vi "Get Primary Key.vi"(8 "error in (no error)":errorcluster, 10 "Table Name Array":string[](array[string]), 11 "ADODB in":refnum<class "ADODB.lvclass">) -> (0 "error out":errorcluster, 1 "PK Found?":bool[](array[boolean]), 2 "Primary Key Array":T1[](array[typedef]), 3 "ADODB out":refnum<class "ADODB.lvclass">)   [LabVIEW 2020, in "ADODB.lvlib" / "ADODB.lvclass"]
uses:
  ADODB.lvclass
  Database Interfaces/Primary Key Info.ctl
  ADODB.lvclass/ADODB.ctl
  ADODB.lvlib
  <vilib>/addons/database/NI_Database_API.lvlib
  Database Interfaces.lvlib
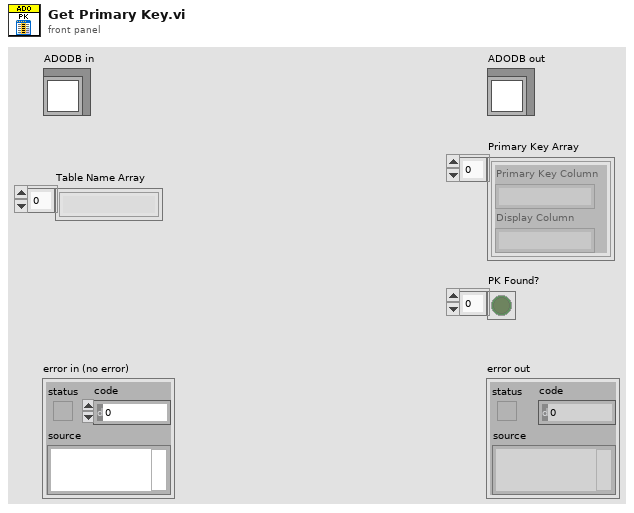
[diagram p1: front panel]
types:
  T1 = typedef "Database Interfaces.lvlib/Primary Key Info.ctl" = cluster{"Primary Key Column":string, "Display Column":string}
  T2 = typedef "NI_Database_API.lvlib/Conn ObjectReference.ctl" = refnum<k1>
  T3 = typedef "NI_Database_API.lvlib/Conn DataMembers.ctl" = cluster{"ADODB._Connection":refnum<k7>, "recordset objects":i32, "command objects":i32}
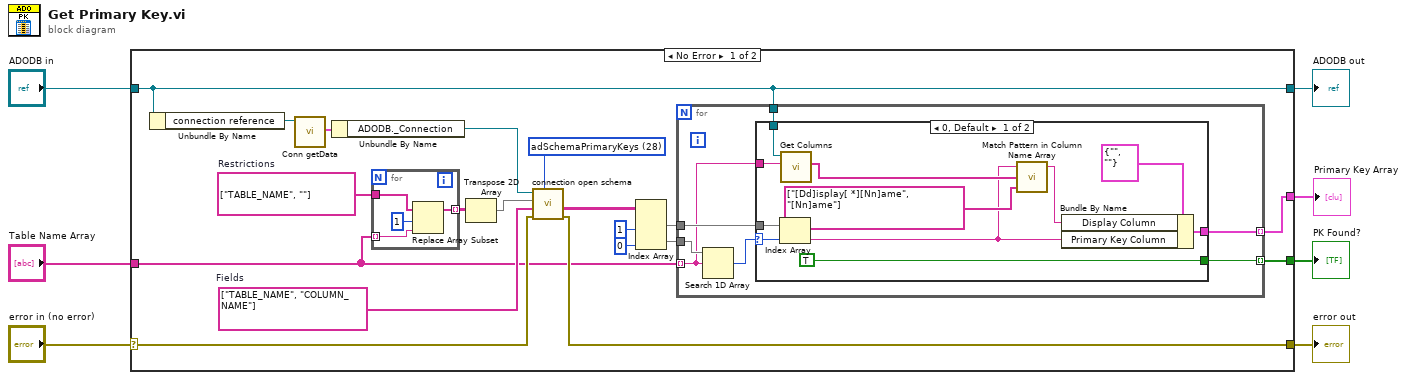
[diagram p0: block diagram]
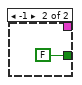
[diagram p2: hidden frame]
diagram:
  n1 = case shown="No Error" "error in (no error)" {
    selector: "error in (no error)" -> [w22 w51]
    tunnel: [w21 w51] -> w6
    tunnel: "ADODB in" -> [w8 w50]
    tunnel: [w8 w50] -> w4
    tunnel: "Table Name Array" -> [w18 _]
    tunnel: [w12 _] -> w1
    tunnel: [w11 _] -> w2
    frame No Error {
      w19 = string[] ["TABLE_NAME", ""]  # Restrictions
      w20 = string[] ["TABLE_NAME", "COLUMN_NAME"]  # Fields
      w23 = 28 items=["adSchemaProviderSpecific"=-1, "adSchemaAsserts"=0, "adSchemaCatalogs"=1, "adSchemaCharacterSets"=2, "adSchemaCollations"=3, "adSchemaColumns"=4, "adSchemaCheckConstraints"=5, "adSchemaConstraintColumnUsage"=6, "adSchemaConstraintTableUsage"=7, "adSchemaKeyColumnUsage"=8, "adSchemaReferentialContraints, adSchemaReferentialConstraints"=9, "adSchemaTableConstraints"=10, "adSchemaColumnsDomainUsage"=11, "adSchemaIndexes"=12, "adSchemaColumnPrivileges"=13, "adSchemaTablePrivileges"=14, "adSchemaUsagePrivileges"=15, "adSchemaProcedures"=16, "adSchemaSchemata"=17, "adSchemaSQLLanguages"=18, "adSchemaStatistics"=19, "adSchemaTables"=20, "adSchemaTranslations"=21, "adSchemaProviderTypes"=22, "adSchemaViews"=23, "adSchemaViewColumnUsage"=24, "adSchemaViewTableUsage"=25, "adSchemaProcedureParameters"=26, "adSchemaForeignKeys"=27, "adSchemaPrimaryKeys"=28, "adSchemaProcedureColumns"=29, "adSchemaDBInfoKeywords"=30, "adSchemaDBInfoLiterals"=31, "adSchemaCubes"=32, "adSchemaDimensions"=33, "adSchemaHierarchies"=34, "adSchemaLevels"=35, "adSchemaMeasures"=36, "adSchemaProperties"=37, "adSchemaMembers"=38, "adSchemaTrustees"=39] ("Schema")
      n2 = Unbundle By Name(w8) -> ("connection reference"=w26:T2)
      n3 = call <vilib>:"Conn getData.vi"("connection reference"=w26) -> ("data"=w25:T3)  [unwired: 3 in, 3 out]
      n4 = Unbundle By Name(w25) -> ("ADODB._Connection"=w24:refnum<k7>)
      n5 = for {
        tunnel: w18 -> [w48] mode=indexing
        tunnel: [w47] -> w10 mode=indexing
        tunnel: w19 -> [w46]
        n6 = Replace Array Subset(array=w46, new element=w48, index=1 ("index (row)")) -> (w47:string[])
      }
      n7 = Transpose 2D Array(2D array=w10) -> (transposed array=w9:string[][])
      n8 = call "connection open schema.vi"("Schema"=w23, "error in (no error)"=w22, "Fields"=w20, "Restrictions"=w9, "ADODB._Connection"=w24) -> ("error out"=w21:errorcluster, "Schema Out"=w17:string[][])  [unwired: 3 in, 2 out]
      n9 = Index Array(array=w17, index (col) #1=1 ("disabled index (col)"), index (col) #2=0 ("index (col)")) -> (element #1=w13:string[], element #2=w14:string[])  [unwired: 2 in]
      n10 = for {
        tunnel: w18 -> [w28] mode=indexing
        tunnel: w14 -> [w33]
        tunnel: w13 -> [w32]
        tunnel: [w27] -> w12 mode=indexing
        tunnel: [w30] -> w11 mode=indexing
        tunnel: w8 -> [w29]
        n11 = Search 1D Array(1D array=w33, element=w28) -> (index of element=w31:i32)  [unwired: 1 in]
        n12 = case shown="0, Default" w31 {
          selector: w31 -> [w44 _]
          tunnel: w32 -> [w43 _]
          tunnel: [TRUE FALSE] -> w30
          tunnel: w29 -> [w41 _]
          tunnel: w28 -> [w40 _]
          tunnel: [w34 _] -> w27
          frame 0, Default {
            n13 = Index Array(array=w43, index=w44) -> (element=w36:string)
            n14 = call-dynamic "Get Columns.vi"("Table Name"=w40, "ADODB in"=w41) -> ("Column Name Array"=w39:string[])  [unwired: 7 in, 2 out]
            n15 = call "Match Pattern in Column Name Array.vi"("Match Pattern Regex"=string[] ["[Dd]isplay[ *][Nn]ame", "[Nn]ame"], "Column Name Array"=w39, "Not Found Name"=w36) -> ("Matching Name"=w35:string)  [unwired: 2 out]
            n16 = Bundle By Name(cluster=T1 {"Primary Key Column"="", "Display Column"=""} ("Primary Key Info"), "Display Column"=w35, "Primary Key Column"=w36) -> (w34:T1)
          }
          frame -1 {
          }
        }
      }
    }
    frame Error {
    }
  }
  "error out" <- w6
  "ADODB out" <- w4
  "PK Found?" <- w2
  "Primary Key Array" <- w1
